vi "BRig_RT__Case_Idle__calc_FPGA_laser.vi"(0 "input_FPGA_ms2count":dbl, 5 "input_Tpeak":dbl, 7 "input_Freq":dbl, 9 "input_Tshutter":dbl) -> (4 "output_laser_Npeak":u32, 6 "output_laser_Nvalley":u32, 8 "output_laser_Nshutter":u32)   [LabVIEW 2014]
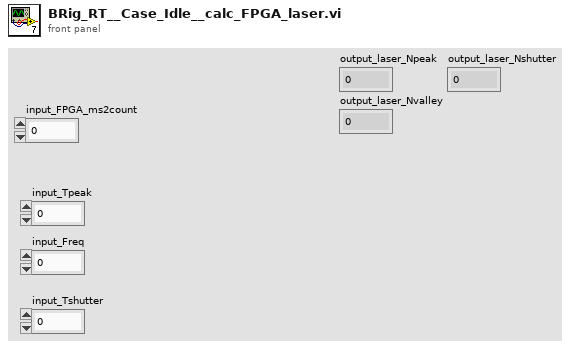
[diagram p1: front panel]
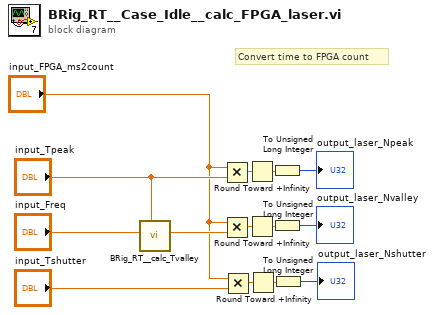
[diagram p0: block diagram]
diagram:
  # "Convert time to FPGA count"
  n1 = call "BRig_RT__calc_Tvalley.vi"("input_peakWidth"="input_Tpeak", "input_freq"="input_Freq") -> ("output_Tvalley"=w6:dbl)  [unwired: 9 in]
  n2 = Multiply(x="input_FPGA_ms2count", y="input_Tpeak") -> (x*y=w9:dbl)
  n3 = Multiply(x="input_FPGA_ms2count", y=w6) -> (x*y=w11:dbl)
  n4 = Multiply(x="input_FPGA_ms2count", y="input_Tshutter") -> (x*y=w12:dbl)
  n5 = Round Toward +Infinity(x=w9) -> (ceil(x): smallest int >= x=w8:dbl)
  n6 = Round Toward +Infinity(x=w11) -> (ceil(x): smallest int >= x=w10:dbl)
  n7 = Round Toward +Infinity(x=w12) -> (ceil(x): smallest int >= x=w13:dbl)
  n8 = To Unsigned Long Integer(number=w8) -> (unsigned 32bit integer=→"output_laser_Npeak":u32)
  n9 = To Unsigned Long Integer(number=w10) -> (unsigned 32bit integer=→"output_laser_Nvalley":u32)
  n10 = To Unsigned Long Integer(number=w13) -> (unsigned 32bit integer=→"output_laser_Nshutter":u32)
